vi "Process_Trigger_Stack.vi"(6 "Add trigger?":bool, 8 "Time":u64, 10 "Last trigger Stack 2":refnum<vi>) -> (0 "Average Trigger":dbl, 2 "Last trigger Stack":refnum<vi>)   [LabVIEW 2010]
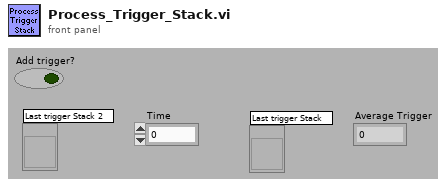
[diagram p1: front panel]
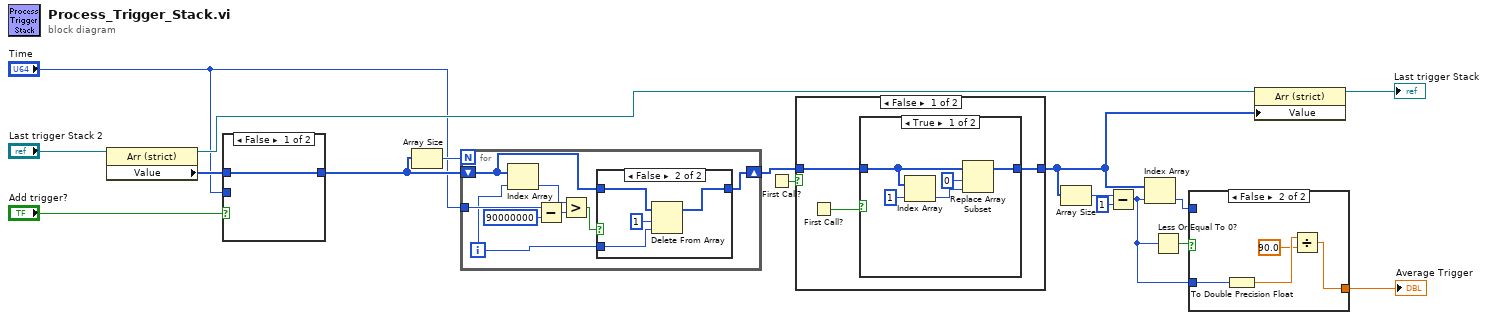
[diagram p0: block diagram]
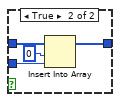
[diagram p2: hidden frame]
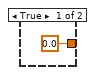
[diagram p3: hidden frame]
diagram:
  n1 = property class="Arr (strict)"(reference="Last trigger Stack 2") -> (reference out=w12:refnum<vi>, "Value"=w3:u64[])  [unwired: 1 in, 1 out]
  n2 = case shown="False" "Add trigger?" {
    tunnel: [w18 w22] -> w4
    tunnel: w3 -> [w18 w21]
    tunnel: "Time" -> [_ w20]
    frame False {
    }
    frame True {
      n3 = Insert Into Array(array=w21, index=0, new element=w20) -> (w22:u64[])
    }
  }
  n4 = Array Size(array=w4) -> (size(s)=w17:i32)
  n5 = for {
    N: w17 -> [_]
    tunnel: "Time" -> [w30]
    shift-right: [w27] -> w14
    shift-left: w4 -> [w23]
    i -> [w25]
    n6 = Index Array(array=w23, index=w25) -> (element=w24:u64)
    n7 = Subtract(x=w30, y=u64 90000000) -> (x-y=w29:u64)
    n8 = Greater?(x=w24, y=w29) -> (0:w28:bool)
    n9 = case shown="False" w28 {
      tunnel: w23 -> [w31 w35]
      tunnel: w25 -> [_ w33]
      tunnel: [w31 w32] -> w27
      frame True {
      }
      frame False {
        n10 = Delete From Array(array=w35, length=1, index=w33) -> (array with subset deleted=w32:u64[])  [unwired: 1 out]
      }
    }
  }
  n11 = First Call?() -> (First Call?: T/F=w10:bool)
  n12 = case shown="False" w10 {
    tunnel: w14 -> [w36 w45]
    tunnel: [w37 w45] -> w11
    frame False {
      n13 = First Call?() -> (First Call?: T/F=w38:bool)
      n14 = case shown="True" w38 {
        tunnel: w36 -> [w41 w44]
        tunnel: [w39 w44] -> w37
        frame True {
          n15 = Index Array(array=w41, index=1) -> (element=w40:u64)
          n16 = Replace Array Subset(array=w41, new element=w40, index=0) -> (w39:u64[])
        }
        frame False {
        }
      }
    }
    frame True {
    }
  }
  n17 = Array Size(array=w11) -> (size(s)=w7:i32)
  n18 = Subtract(x=w7, y=1) -> (x-y=w16:i32)
  n19 = Index Array(array=w11, index=w16) -> (element=w8:u64)
  n20 = Less Or Equal To 0?(x=w16) -> (x <= 0?=w15:bool)
  n21 = case shown="False" w15 {
    tunnel: w16 -> [_ w49]
    tunnel: w8 -> [_ _]
    tunnel: [0.0 w48] -> w9
    frame True {
    }
    frame False {
      n22 = To Double Precision Float(number=w49) -> (double precision float=w50:dbl)
      n23 = Divide(x=w50, y=90.0) -> (x/y=w48:dbl)
    }
  }
  "Average Trigger" <- w9
  n24 = property class="Arr (strict)"(reference=w12, "Value"=w11) -> (reference out=→"Last trigger Stack":refnum<vi>)  [unwired: 1 in, 1 out]
